vi "NI6071E.evt call Stop DAQ.vi"(0 "i ref in":refnum<vi>, 2 "Client":string, 3 "Client timeout (10000)":i32=10000, 5 "error in (no error)":errorcluster) -> (14 "i ref out":refnum<vi>, 19 "error out":errorcluster)   [LabVIEW 2014, in "NI6071E.lvlib"]
doc: "This VI asks for an event by a simple call"
uses:
  NI6071E.lvlib
  NI6071ECommand.ctl
  CSCore/CSSystem/CoreLib/CoreLib.int 2 byte array.vi
  CSCore/BaseProcess/BaseProcess.lvlib
  CSCore/CSSystem/CoreLib/CoreLib.lvlib
panel:
  in  "NI6071E Command":T1=enum."StopDAQ"
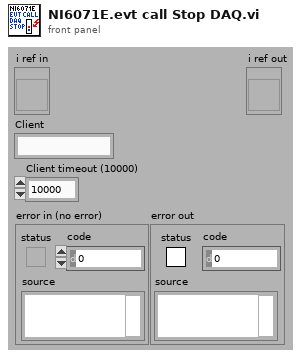
[diagram p1: front panel]
types:
  T1 = typedef "NI6071E.lvlib/NI6071ECommand.ctl" = enum16{"Ping", "Reset", "ConfigureDAQ", "StartDAQ", "StopDAQ", "GetDAQStatus", "ReadData", "SaveData", "CloseConnection"}
  T2 = typedef "CoreDefs.rawDataType.ctl" = i8[]
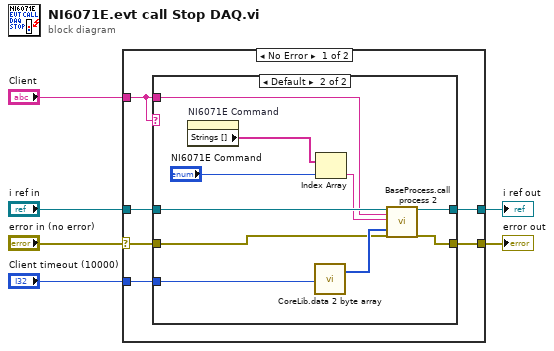
[diagram p0: block diagram]
diagram:
  n1 = case shown="No Error" "error in (no error)" {
    selector: "error in (no error)" -> [w8 w25]
    tunnel: [w12 w25] -> w6
    tunnel: "i ref in" -> [w11 w26]
    tunnel: "Client" -> [w7 _]
    tunnel: [w10 w26] -> w3
    tunnel: "Client timeout (10000)" -> [w9 _]
    frame No Error {
      n2 = case shown="Default" w7 {
        tunnel: [w13 w24] -> w12
        tunnel: w11 -> [w14 w23]
        tunnel: w7 -> [_ w22]
        tunnel: [w14 w21] -> w10
        tunnel: w9 -> [_ w16]
        tunnel: w8 -> [w13 w15]
        frame "N/A" {
        }
        frame Default {
          n3 = property on="NI6071E Command" class="Enum (strict)"() -> ("Strings []"=w19:string[])  [unwired: 2 in, 2 out]
          n4 = call-poly "CoreLib.data 2 byte array.vi"("i32"=w16) -> ("byteArray out"=w17:T2)  [unwired: 18 in]
          n5 = Index Array(array=w19, index="NI6071E Command") -> (element=w18:string)
          n6 = call "BaseProcess.call process 2.vi"("i ref in"=w23, "Object"=w22, "Selector"=w18, "Data"=w17, "error in (no error)"=w15) -> ("i ref out"=w21:refnum<vi>, "error out"=w24:errorcluster)  [unwired: 13 in]
        }
      }
    }
    frame Error {
    }
  }
  "error out" <- w6
  "i ref out" <- w3
